vi "SaveToDisk.vi"(0 "Session Handle in":T1, 11 "error in (no error)":errorcluster) -> (4 "Session Handle out":T1, 15 "error out":errorcluster)   [LabVIEW 2020, in "TSS.lvlib" / "VariableContainer.lvclass"]
uses:
  VariableContainer.lvclass
  Typedefs/Session Handle.ctl
  VariableContainer.lvclass/VariableContainer.ctl
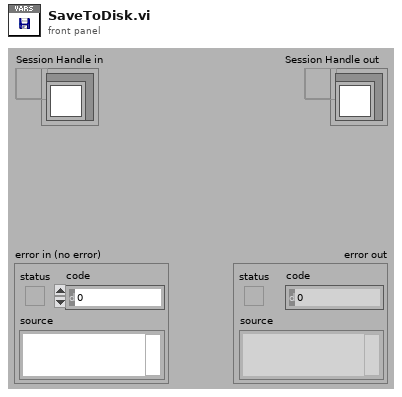
[diagram p1: front panel]
types:
  T1 = typedef "TSS.lvlib/VariableContainer.lvclass/Session Handle.ctl" = refnum<data-value>
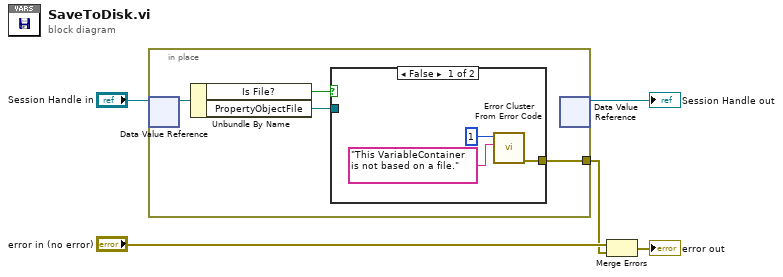
[diagram p0: block diagram]
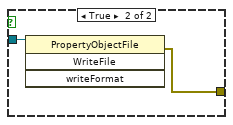
[diagram p2: hidden frame]
diagram:
  n1 = in-place {
    in-place-border: [w6] -> w2
    n2 = in-place-dvr #1("Session Handle in") -> (w9:refnum<class "VariableContainer.lvclass">)  [unwired: 1 out]
    n3 = Unbundle By Name(w9) -> ("Is File?"=w8:bool, "PropertyObjectFile"=w7:refnum<k7>)
    n4 = case shown="False" w8 {
      tunnel: w7 -> [_ w14]
      tunnel: [w12 w13] -> w6
      frame False {
        n5 = call <vilib>:"Error Cluster From Error Code.vi"("error message (\"\")"="This VariableContainer is not based on a file." ("error message (\"\")"), "error code (0)"=1) -> ("error out"=w12:errorcluster)  [unwired: 7 in]
      }
      frame True {
        n6 = invoke class="PropertyObjectFile" method="WriteFile"(reference=w14) -> (error out=w13:errorcluster)  [unwired: 3 in, 3 out]
      }
    }
    n7 = in-place-dvr #1() -> (→"Session Handle out":T1)  [unwired: 1 in, 1 out]
  }
  n8 = Merge Errors("error in (no error)", w2) -> (→"error out":errorcluster)
